vi "DirettoreReadBack.vi"(0 "FPGAReference":refnum<k20>) -> (4 "MatrixOut":i16[](array[numeric]), 15 "ErrorOut":errorcluster)   [LabVIEW 2012]
uses:
  <vilib>/rvi/interface/nirviMethod/nirviMethod.xnode
  <vilib>/FPGAPlugInAG/Dynamic/niLvFpga_ReadFifo_Dynamic.vi
  <vilib>/rvi/errors/niLvFpgaMergeErrorWithErrorCode.vi
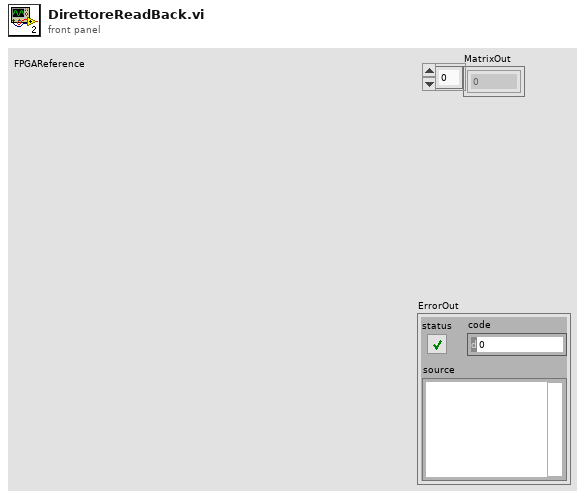
[diagram p1: front panel]
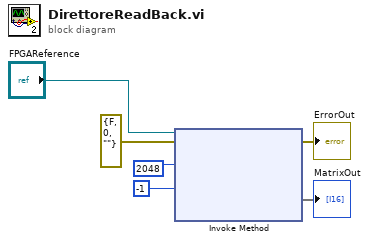
[diagram p0: block diagram]
diagram:
  n1 = xnode "Invoke Method"("FPGA VI Reference In"="FPGAReference", "error in"=errorcluster {"status"=FALSE, "code"=0, "source"=""} ("error out"), "Number of Elements"=u32 2048, "Timeout (ms)"=-1) -> ("error out"=→"ErrorOut":errorcluster, "Data"=→"MatrixOut":void[])  [unwired: 2 out]
